vi "Get Data Pointers in Profile Structure.vi"(0 "Profile Info":T1, 11 "error in (no error)":errorcluster caption="エラー入力 (エラーなし)") -> (4 "Height Profile Pointer Index":u32, 6 "Luminance Profile Pointer Index":u32, 8 "Footer Pointer Index":u32, 10 "Data Num of Raw Profile Structure":u32, 15 "error out":errorcluster caption="エラー出力")   [LabVIEW 2020, in "KEYENCE LJ-X8000A.lvlib"]
uses:
  KEYENCE LJ-X8000A.lvlib
  Public/Clusters/Profile Info.ctl
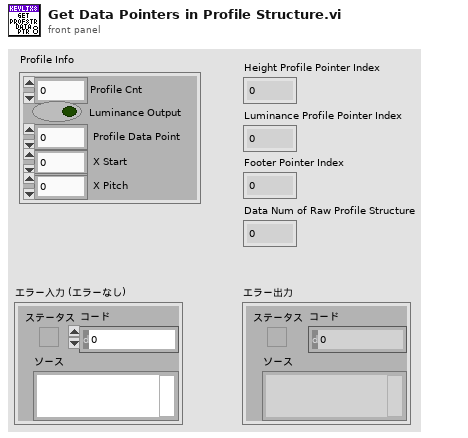
[diagram p1: front panel]
types:
  T1 = typedef "KEYENCE LJ-X8000A.lvlib/Profile Info.ctl" = cluster{"Profile Cnt":u8, "Luminance Output":bool, " Profile Data Point":u16, " X Start":i32, " X Pitch":i32}
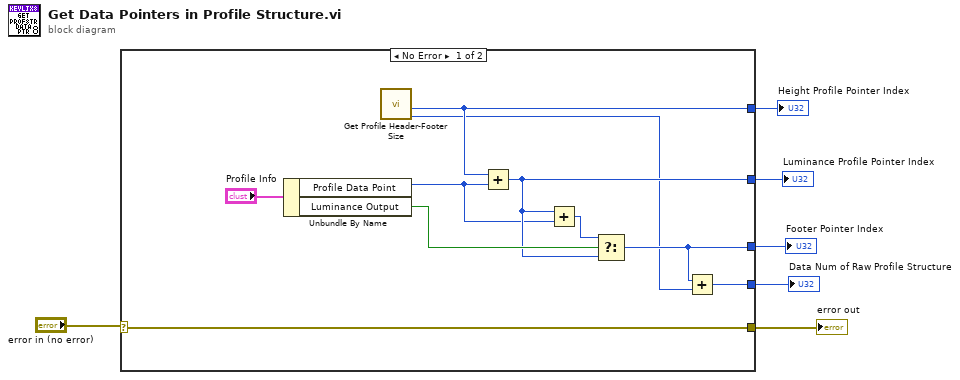
[diagram p0: block diagram]
diagram:
  n1 = case shown="No Error" "error in (no error)" {
    selector: "error in (no error)" -> [w11 w17]
    tunnel: [w15 _] -> w6
    tunnel: [w12 _] -> w5
    tunnel: [w10 _] -> w4
    tunnel: [w11 w17] -> w2
    tunnel: [w8 _] -> w1
    frame No Error {
      n2 = Unbundle By Name("Profile Info") -> ("Profile Data Point"=w7:u16, "Luminance Output"=w14:bool)
      n3 = call "Get Profile Header-Footer Size.vi"() -> ("Footer Size(DWORD)"=w9:u32, "Header Size(DWORD)"=w15:u32)  [unwired: 8 in, 2 out]
      n4 = Add(x=w15, y=w7) -> (x+y=w12:u32)
      n5 = Add(x=w12, y=w7) -> (x+y=w13:u32)
      n6 = Select(t=w13, s=w14, f=w12) -> (s? t:f=w10:u32)
      n7 = Add(x=w10, y=w9) -> (x+y=w8:u32)
    }
    frame Error {
    }
  }
  "Height Profile Pointer Index" <- w6
  "Footer Pointer Index" <- w4
  "Luminance Profile Pointer Index" <- w5
  "error out" <- w2
  "Data Num of Raw Profile Structure" <- w1
